vi "Initilisation_AOTF.vi"(5 "error in":errorcluster) -> (19 "error out":errorcluster)   [LabVIEW 2013]
uses:
  Variables/GlobalGetAOTFOnOff.vi
  Variables/AOTFStatus.vi
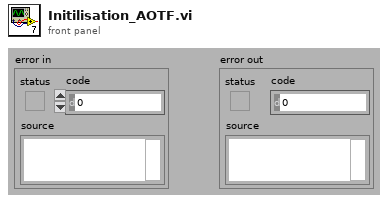
[diagram p1: front panel]
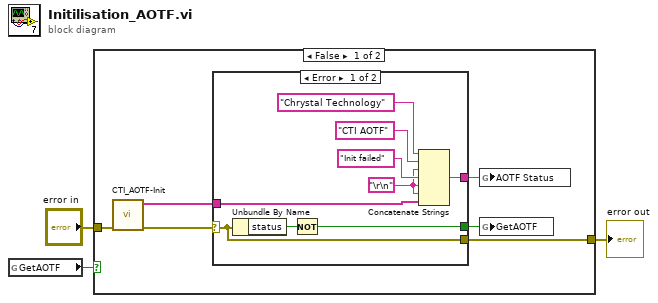
[diagram p0: block diagram]
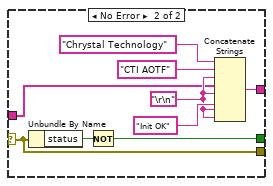
[diagram p2: hidden frame]
diagram:
  n1 = global read "GlobalGetAOTFOnOff.vi" "GetAOTF"() -> (w1:bool)
  n2 = case shown="False" w1 {
    tunnel: [w6 w28] -> w3
    tunnel: "error in" -> [w9 w28]
    frame False {
      n3 = call "CTI_AOTF-Init.vi"("error in"=w9) -> ("error out"=w5:errorcluster, "Config Out"=w8:string[])  [unwired: 9 in]
      n4 = case shown="Error" w5 {
        selector: w5 -> [w12 w23]
        tunnel: w8 -> [w10 w19]
        tunnel: [w16 w24] -> w7
        tunnel: [w12 w23] -> w6
        tunnel: [w13 w21] -> w4
        frame Error {
          w15 = "\r\n"
          n5 = Unbundle By Name(w12) -> ("status"=w14:bool)
          n6 = Not(x=w14) -> (.not. x?=w13:bool)
          n7 = Concatenate Strings("Chrystal Technology" ("string"), "CTI AOTF" ("string"), w15, "Init failed" ("string"), w15, w15, w10) -> (w16:string)
        }
        frame No Error {
          w25 = "\r\n"
          n8 = Unbundle By Name(w23) -> ("status"=w22:bool)
          n9 = Not(x=w22) -> (.not. x?=w21:bool)
          n10 = Concatenate Strings("Chrystal Technology" ("string"), "CTI AOTF" ("string"), w25, w19, w25, "Init OK" ("string"), w25, w25) -> (w24:string)
        }
      }
      n11 = global write "AOTFStatus.vi" "AOTF Status"(w7) -> ()
      n12 = global write "GlobalGetAOTFOnOff.vi" "GetAOTF"(w4) -> ()
    }
    frame True {
    }
  }
  "error out" <- w3
